vi "All Entities.vi"(8 "error in (no error)":errorcluster, 11 "EntityPersistMap in":refnum<class "EntityPersistMap.lvclass">) -> (0 "error out":errorcluster, 2 "All Entities":T1(array[cluster]))   [LabVIEW 2020, in "Conditum SQLite.lvlib" / "EntityPersistMap.lvclass"]
uses:
  EntityPersistMap.lvclass
  EntityPersistMap.lvclass/EntityPersistMap.ctl
  <vilib>/IlluminatedG/IG Conditum Base/Conditum/Entity/Entity.lvclass
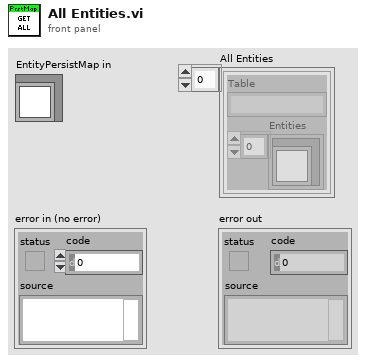
[diagram p1: front panel]
types:
  T1 = cluster{"Table":string, "Entities":refnum<class "Entity.lvclass">[]}[]
  T2 = typedef "Conditum.lvlib/Entity ID.ctl" = i64
  T3 = map{string, map{T2, refnum<class "Entity.lvclass">}}
  T4 = cluster{"Table":string, refnum<class "Entity.lvclass">[]}
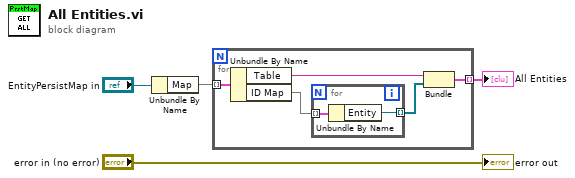
[diagram p0: block diagram]
diagram:
  n1 = Unbundle By Name("EntityPersistMap in") -> ("Map"=w2:T3)
  n2 = for {
    tunnel: w2 -> [w9] mode=indexing
    tunnel: [w5] -> w1 mode=indexing
    n3 = Unbundle By Name(w9) -> ("Table"=w7:string, "ID Map"=w8:map{T2, refnum<class "Entity.lvclass">})
    n4 = for {
      tunnel: w8 -> [w11] mode=indexing
      tunnel: [w10] -> w6 mode=indexing
      n5 = Unbundle By Name(w11) -> ("Entity"=w10:refnum<class "Entity.lvclass">)
    }
    n6 = Bundle("Table"=w7, w6) -> (w5:T4)  [unwired: 1 in]
  }
  "All Entities" <- w1
  "error out" <- "error in (no error)"
